vi "Init.vi"(8 "error in (no error)":errorcluster, 10 "Instrument Ref":variant, 11 "niPower in":refnum<class "NI DC Power.lvclass">) -> (0 "error out":errorcluster, 2 "Found?":bool, 3 "niPower out":refnum<class "NI DC Power.lvclass">)   [LabVIEW 2025, in "Power Supply.lvlib" / "NI DC Power.lvclass"]
uses:
  NI DC Power.lvclass
  C:/Working copy/tss/Plugin/Engines/Power Supply/PS Instrument/Power Supply Instrument.lvclass
  Users/Public/Documents/Sandia National Labs/TSS Plugin/Abstract Engine.lvlibp/Instrument configuration/Instrument configuration.lvclass
  NI DC Power.lvclass/NI DC Power.ctl
  Users/Public/Documents/Sandia National Labs/TSS Plugin/Abstract Engine.lvlibp/Instrument configuration/Read Instrument Setting.vi
  Users/Public/Documents/Sandia National Labs/TSS Plugin/CEF.lvlibp/serializable configuration/CEF_serializable configuration.lvclass
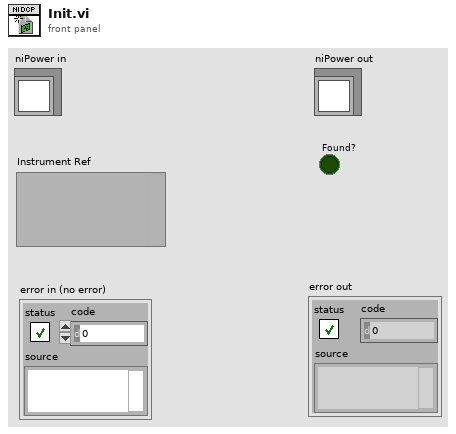
[diagram p1: front panel]
types:
  T1 = typedef "Abstract Engine.lvlibp/Instrument configuration.lvclass/Default Instrument.ctl" = cluster{"Type":string, "Address":string, "SW Alias":string, "Description":string, "Enabled":bool}
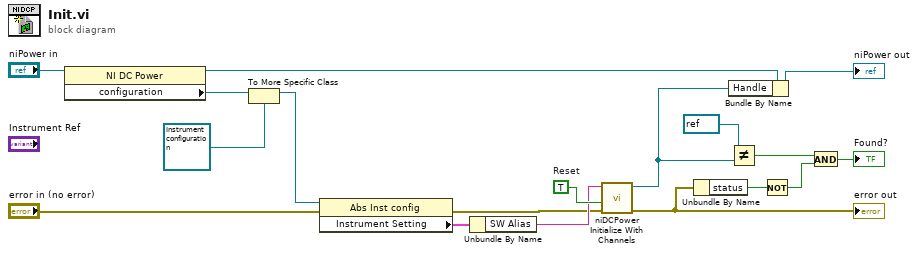
[diagram p0: block diagram]
diagram:
  w17 = TRUE  # Reset
  n1 = property class="NI DC Power"(reference="niPower in") -> (reference out=w12:refnum<class "NI DC Power.lvclass">, "configuration"=w11:refnum<class "CEF_serializable configuration.lvclass">)  [unwired: 1 in, 1 out]
  n2 = To More Specific Class(target class=refnum<class "Instrument configuration.lvclass"> refnum ("Abstract PlugIn.lvlibp:Instrument configuration"), reference=w11) -> (specific class reference=w10:refnum<class "Instrument configuration.lvclass">)  [unwired: 1 in, 1 out]
  n3 = property class="Abs Inst config"(reference=w10, error in="error in (no error)") -> (error out=w8:errorcluster, "Instrument Setting"=w1:T1)  [unwired: 1 out]
  n4 = Unbundle By Name(w1) -> ("SW Alias"=w13:string)
  n5 = call <instrlib>:"niDCPower Initialize With Channels.vi"("error in (no error)"=w8, "reset (false)"=w17, "resource name"=w13) -> ("error out"=w6:errorcluster, "instrument handle out"=w16:refnum<k15>)  [unwired: 7 in]
  "error out" <- w6
  n6 = Unbundle By Name(w6) -> ("status"=w7:bool)
  n7 = Bundle By Name(cluster=w12, "Handle"=w16) -> (→"niPower out":refnum<class "NI DC Power.lvclass">)
  n8 = Not Equal?(x=refnum<k15> refnum, y=w16) -> (x != y?=w4:bool)
  n9 = Not(x=w7) -> (.not. x?=w5:bool)
  n10 = And(x=w4, y=w5) -> (x .and. y?=→"Found?":bool)
